vi "GetDepsList.vi"(8 "error in (no error)":errorcluster, 10 "Library / Class Name":string, 11 "WorkSpace / Repo path":path) -> (0 "error out":errorcluster, 2 "Indirect Dependency []":string[](array[string]), 3 "Direct Dependency []":string[](array[string]))   [LabVIEW 2019, in "Hawkeye.lvlib"]
uses:
  Hawkeye.lvlib
  799445fe-521b-4170-8b29-c1a997ec6070.vi
  <userlib>/_OpenG.lib/file/file.llb/File Exists - Scalar__ogtk.vi
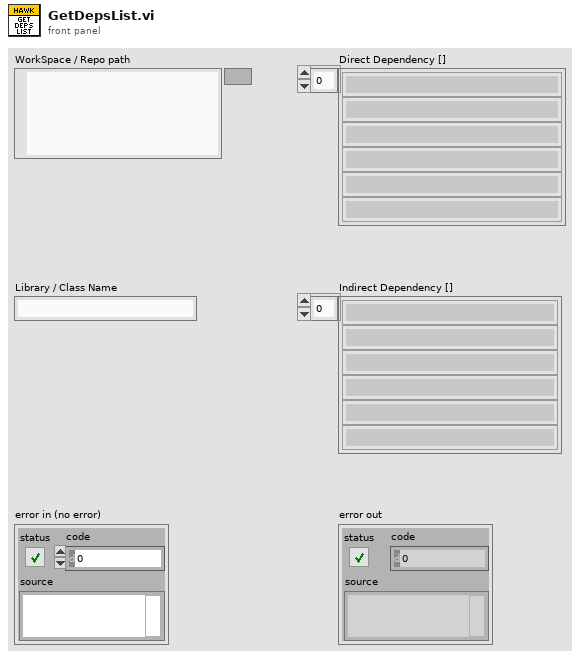
[diagram p1: front panel]
types:
  T1 = enum16{"open", "replace", "create", "open or create", "replace or create", "replace or create with confirmation"}
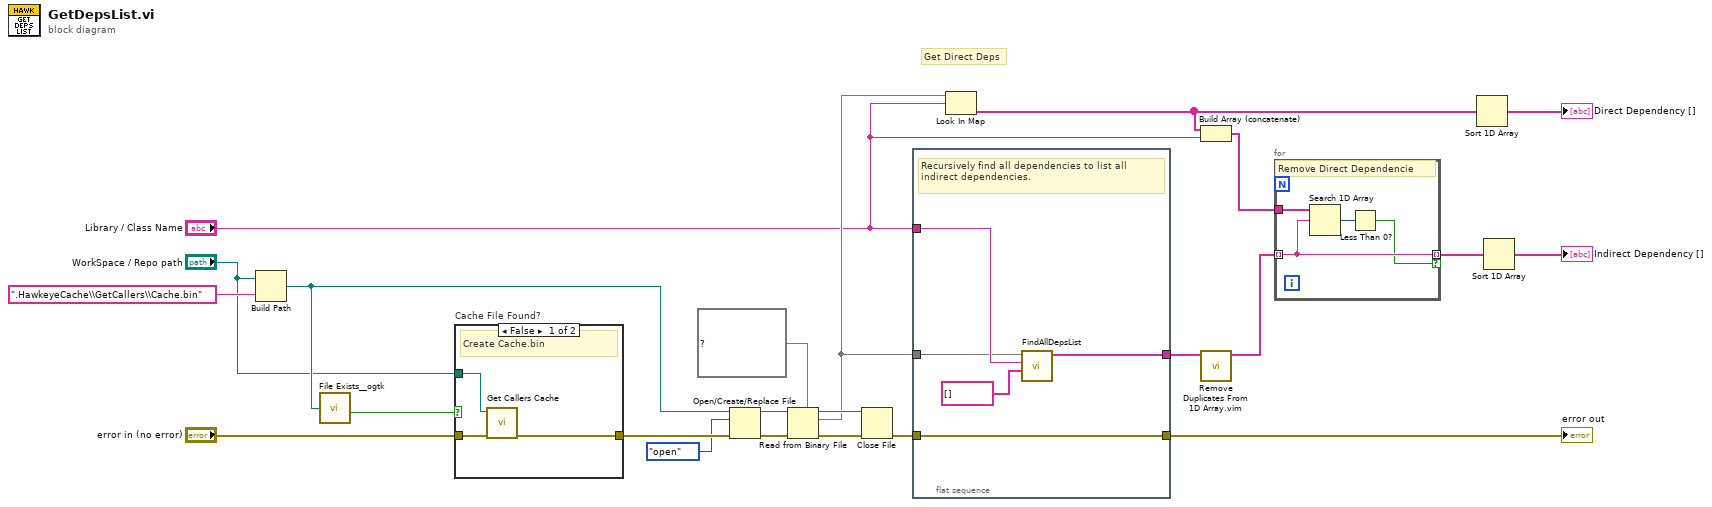
[diagram p0: block diagram]
diagram:
  # "Get Direct Deps"
  n1 = Build Path(base path="WorkSpace / Repo path", name or relative path=".HawkeyeCache\\GetCallers\\Cache.bin") -> (appended path=w3:path)
  n2 = call-poly <userlib>:"File Exists__ogtk.vi"("file path"=w3) -> ("exists"=w4:bool)  [unwired: 6 in, 1 out]
  n3 = case "Cache File Found?" shown="False" w4 {
    tunnel: "error in (no error)" -> [w26 w27]
    tunnel: [w25 w27] -> w5
    tunnel: "WorkSpace / Repo path" -> [w24 _]
    frame False {
      # "Create Cache.bin"
      n4 = call "Get Callers Cache.vi"("error in (no error)"=w26, "WorkSpace / Repo path"=w24) -> ("error out"=w25:errorcluster)  [unwired: 8 in, 1 out]
    }
    frame True {
    }
  }
  n5 = Open/Create/Replace File(file path (use dialog)=w3, error in=w5, operation (0:open)=T1."open") -> (refnum out=w22:refnum<file>, error out=w19:errorcluster)  [unwired: 3 in, 1 out]
  n6 = Read from Binary File(5:map{string, string[]} {} ("Dependency Map"), 8:w19, 11:w22) -> (0:w20:errorcluster, 2:w14:map{string, string[]}, 3:w21:refnum<file>)  [unwired: 3 in, 1 out]
  n7 = Close File(refnum=w21, error in=w20) -> (error out=w15:errorcluster)  [unwired: 1 out]
  n8 = flat-sequence {
    tunnel: "Library / Class Name" -> [w32]
    tunnel: [w30] -> w23
    tunnel: w14 -> [w29]
    tunnel: [w28] -> w16
    tunnel: w15 -> [w28]
    frame #0 {
      # "Recursively find all dependencies to list all indirect dependencies."
      n9 = call "FindAllDepsList.vi"("Dependency List [] In"=string[] [] ("Dependency"), "Current Deps to Check"=w32, "Dependency Map"=w29) -> ("Dependency List [] Out"=w30:string[])  [unwired: 8 in]
    }
  }
  n10 = Look In Map(map=w14, key="Library / Class Name") -> (value=w9:string[])  [unwired: 1 in, 1 out]
  n11 = Build Array (concatenate)(w9, "Library / Class Name") -> (w11:string[])
  n12 = call "Remove Duplicates From 1D Array.vim"("array"=w23) -> ("array with duplicates removed"=w12:string[])  [unwired: 10 in]
  n13 = for {
    tunnel: w12 -> [w35] mode=indexing
    tunnel: w11 -> [w36]
    tunnel: [w35] -> w10 mode=indexing if=w33
    # "Remove Direct Dependencie"
    n14 = Search 1D Array(1D array=w36, element=w35) -> (index of element=w34:i32)  [unwired: 1 in]
    n15 = Less Than 0?(x=w34) -> (x < 0?=w33:bool)
  }
  n16 = Sort 1D Array(array=w9) -> (sorted array=→"Direct Dependency []":string[])
  n17 = Sort 1D Array(array=w10) -> (sorted array=→"Indirect Dependency []":string[])
  "error out" <- w16
